vi "Demo_terminal.vi"() -> ()   [LabVIEW 2017]
panel:
  out "Err no":i16
  out "Err text":string
  out "RX error":bool
  out "Connected":bool
  out "error out":errorcluster
  in  "Exit":bool
  in  "Send":bool
  in  "CMD":string="*IDN?"
  out "Response":string
  in  "VISA resource name":refnum<visa-resource-name>
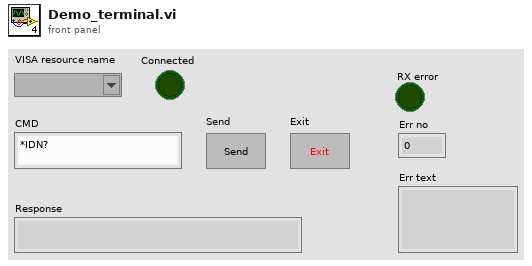
[diagram p1: front panel]
types:
  T1 = cluster{"VISA resource name out":refnum<visa-resource-name>, "error out":errorcluster}
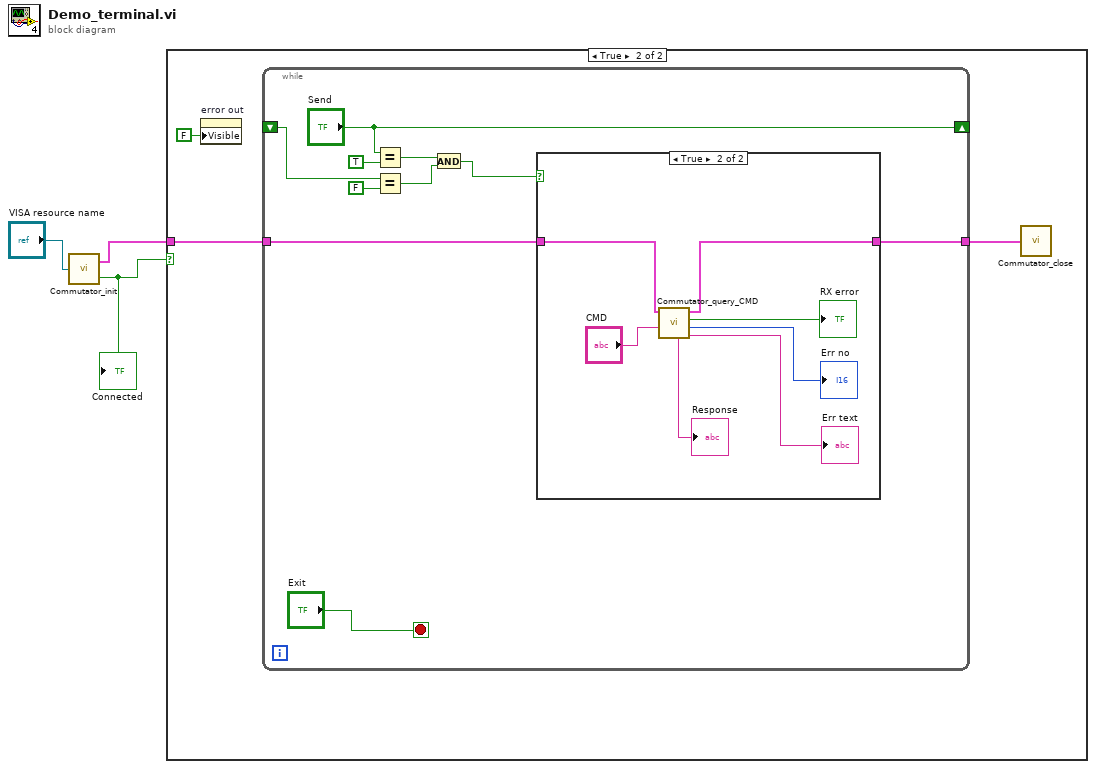
[diagram p0: block diagram]
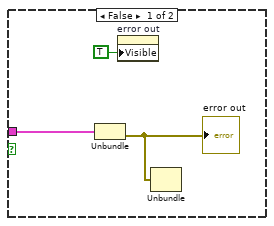
[diagram p2: hidden frame]
diagram:
  n1 = call "Commutator_init.vi"("VISA resource name"="VISA resource name") -> ("status"=w1:bool, "VISA out"=w3:T1)  [unwired: 2 in]
  "Connected" <- w1
  n2 = case shown="True" w1 {
    tunnel: w3 -> [w6 w8]
    frame False {
      n3 = Unbundle(w6) -> ("error out"=w5:errorcluster)  [unwired: 1 out]
      "error out" <- w5
      n4 = property on="error out" class="Clust (strict)"("Visible"=TRUE) -> ()  [unwired: 2 in, 2 out]
      n5 = Unbundle(w5) -> ()  [unwired: 3 out]
    }
    frame True {
      n6 = property on="error out" class="Clust (strict)"("Visible"=FALSE) -> ()  [unwired: 2 in, 2 out]
      n7 = while {
        shift-right: ["Send"] -> _
        shift-left: _ -> [w14]
        tunnel: w8 -> [w11]
        tunnel: [w10] -> w9
        stop <- "Exit" stop-if-true
        n8 = Equal?(x="Send", y=TRUE) -> (x = y?=w18:bool)
        n9 = Equal?(x=w14, y=FALSE) -> (x = y?=w17:bool)
        n10 = And(x=w18, y=w17) -> (x .and. y?=w12:bool)
        n11 = case shown="True" w12 {
          tunnel: w11 -> [w20 w27]
          tunnel: [w20 w25] -> w10
          frame False {
          }
          frame True {
            n12 = call "Commutator_query_CMD.vi"("CMD"="CMD", "VISA in"=w27) -> ("Err text"=→"Err text":string, "Err no"=→"Err no":i16, "RX error"=→"RX error":bool, "VISA out"=w25:T1, "Response"=→"Response":string)  [unwired: 5 in]
          }
        }
      }
      n13 = call "Commutator_close.vi"("VISA in"=w9) -> ()  [unwired: 1 out]
    }
  }
